vi "UTILITY JKI Loop Speed Adjust.vi"(4 "Current Rate":dbl, 6 "Scan Rate Less Than 0.2s":bool, 9 "K(7) - Adjustment Factor":dbl=0.3, 10 "Scan Rate Target":dbl, 11 "Previous Value":dbl) -> (3 "New Time":dbl)   [LabVIEW 2020]
panel:
  out "Going into Correction Loop?":bool
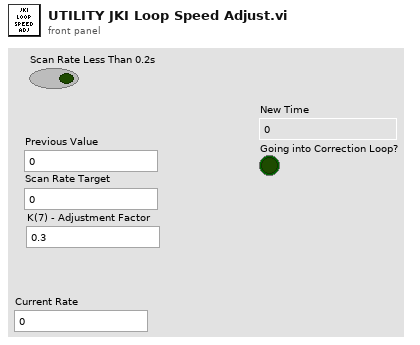
[diagram p1: front panel]
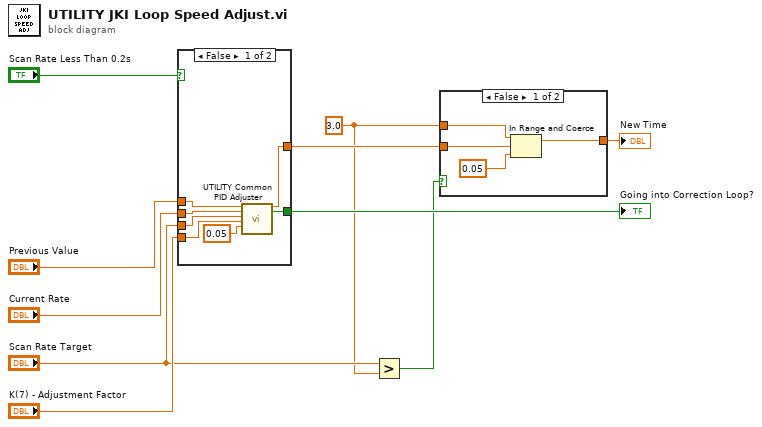
[diagram p0: block diagram]
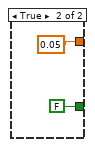
[diagram p3: hidden frame]
diagram:
  w2 = 3.0 ("upper limit")
  n1 = case shown="False" "Scan Rate Less Than 0.2s" {
    tunnel: [w17 0.05 ("New GPM Value")] -> w8
    tunnel: "Previous Value" -> [w16 _]
    tunnel: "Scan Rate Target" -> [w15 _]
    tunnel: "Current Rate" -> [w14 _]
    tunnel: "K(7) - Adjustment Factor" -> [w12 _]
    tunnel: [w11 FALSE ("Going into Correction Loop?")] -> w4
    frame False {
      n2 = call "UTILITY Common PID Adjuster.vi"("Previous Value"=w16, "Current Rate"=w14, "Scan Rate Target"=w15, "K(7) - Adjustment Factor"=w12, "ErrorPassBand(%)"=0.05) -> ("New MicroAmp"=w17:dbl, "Going into Correction Loop?"=w11:bool)  [unwired: 11 in, 2 out]
    }
    frame True {
    }
  }
  "Going into Correction Loop?" <- w4
  n3 = Greater?(x="Scan Rate Target", y=w2) -> (0:w1:bool)
  n4 = case shown="False" w1 {
    tunnel: [w23 w24] -> w9
    tunnel: w8 -> [w22 w24]
    tunnel: w2 -> [w20 _]
    frame False {
      n5 = In Range and Coerce(upper limit=w20, x=w22, lower limit=0.05) -> (coerced(x)=w23:dbl)  [unwired: 1 out]
    }
    frame True {
    }
  }
  "New Time" <- w9
